vi "NXT-CAM-Remote.vi"() -> ()   [LabVIEW 2009]
uses:
  <vilib>/NXT/Subs/LVHSConnector.ctl
  <vilib>/NXT/Block Support/NXT_InputPort.ctl
  <vilib>/NXT/Dual Mode Library/Display/NXT_Rect.ctl
panel:
  in  "Tracking Mode":u8(ring) items=["Disable Tracking", "Get First Object", "Get n th Object", "Enable Tracking", "Sort Objects  by size", "Sort Objects  by Colors", "Illumination on ", "Illumination Off", "Write Colormap", "Read Colormap", "Line tracking mode", "Object Tracking mode"]
  in  "Object Number to Track":u8 format="%x"
  in  "Input Port":T1 caption="Port (Port 4)" items=["Port 1", "Port 2", "Port 3", "Port 4"]
  in  "Height":i32
  in  "Width":i32
  in  "Left":i32
  in  "Bottom":i32
  in  "NXT":T2={"error"={"status"=FALSE, "code"=0, "source"=""}, "address"="", "NXT #"=-1, "Show Error"=TRUE}
  out "Total Objects":u8=8
  out "X Upper Left":u8=108
  out "X Lower Right":u8=155
  out "Y Lower Right":u8=113
  out "Y Upper Left":u8=80
  out "Color":u8=1
  out "NXT dup":T2={"error"={"status"=FALSE, "code"=0, "source"=""}, "address"="", "NXT #"=-1, "Show Error"=TRUE} caption="NXT"
  out "Status \n(boolean)":bool
  # "mindsensors.com\nCopyright (c) 2009 by mindsensors.com\nEmail: info (<at>) mindsensors (<dot>) com\n\nThis program is free software. You can redistribute it and/or modify\nit under the terms of the GNU General Public License as published by\nthe Free Software Foundation; version 3 of the License.\nRead the license at: http://www.gnu.org/licenses/gpl.txt"
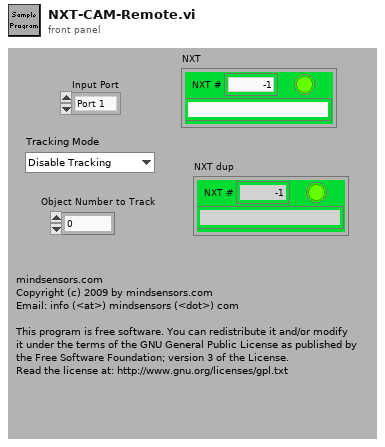
[diagram p1: front panel]
types:
  T1 = typedef "NXT_InputPort.ctl" = u8
  T2 = typedef "LVHSConnector.ctl" = cluster{"error":errorcluster, "address":string, "NXT #":i32, "Show Error":bool}
  T3 = typedef "NXT_Rect.ctl" = cluster{"Left":i16, "Bottom":i16, "Width":i16, "Height":i16}
  T4 = cluster{"Bottom":i32, "Left":i32, "Width":i32, "Height":i32}
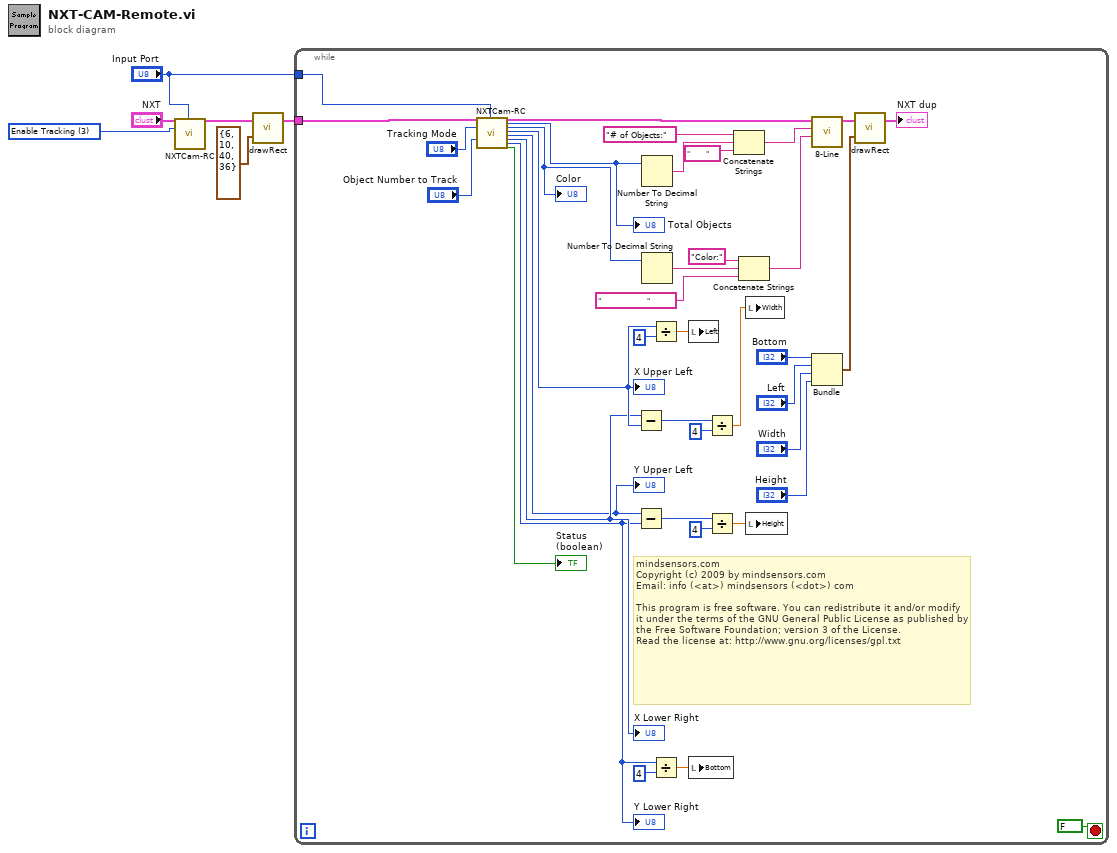
[diagram p0: block diagram]
diagram:
  w1 = u8 3 items=["Disable Tracking", "Get First Object", "Get n th Object", "Enable Tracking", "Sort Objects  by size", "Sort Objects  by Colors", "Illumination on ", "Illumination Off", "Write Colormap", "Read Colormap", "Line tracking mode", "Object Tracking mode"] ("Tracking Mode")
  n1 = call "NXTCam-RC.vi"("NXT"="NXT", "Tracking Mode"=w1, "Input Port"="Input Port") -> ("NXT dup"=w4:T2)  [unwired: 17 in, 7 out]
  n2 = call <vilib>:"drawRect.vi"("Rect Parameters"=T3 {"Left"=6, "Bottom"=10, "Width"=40, "Height"=36}, "NXT"=w4) -> ("NXT"=w3:T2)  [unwired: 2 in]
  n3 = while {
    tunnel: w3 -> [w44]
    tunnel: "Input Port" -> [w43]
    stop <- FALSE stop-if-true
    # "mindsensors.com\nCopyright (c) 2009 by mindsensors.com\nEmail: info (<at>) mindsensors (<dot>) com\n\nThis program is free software. You can redistribute it and/or modify\nit under the terms of the GNU General Public License as published by\nthe Free Software Foundation; version 3 of the License.\nRead the license at: http://www.gnu.org/licenses/gpl.txt"
    n4 = call "NXTCam-RC.vi"("NXT"=w44, "Tracking Mode"="Tracking Mode", "Object Number to Track"="Object Number to Track", "Input Port"=w43) -> ("NXT dup"=w19:T2, "Total Tracked Objects"=w15:u8, "Color"=w14:u8, "X Upper Left"=w13:u8, "Y Upper Left"=w11:u8, "X Lower Right"=w12:u8, "Y Lower Right"=w10:u8, "Status (boolean)"=→"Status \n(boolean)":bool)  [unwired: 16 in]
    "Total Objects" <- w15
    "X Upper Left" <- w13
    "X Lower Right" <- w12
    "Y Lower Right" <- w10
    "Y Upper Left" <- w11
    "Color" <- w14
    n5 = Subtract(x=w12, y=w13) -> (x-y=w23:u8)
    n6 = Subtract(x=w11, y=w10) -> (x-y=w20:u8)
    n7 = Number To Decimal String(number=w15) -> (decimal integer string=w37:string)  [unwired: 1 in]
    n8 = Number To Decimal String(number=w14) -> (decimal integer string=w39:string)  [unwired: 1 in]
    n9 = Divide(x=w13, y=4) -> (x/y=w26:dbl)
    n10 = Divide(x=w10, y=4) -> (x/y=w27:dbl)
    n11 = local write "Left"(w26) -> ()
    n12 = local write "Bottom"(w27) -> ()
    n13 = Divide(x=w23, y=4) -> (x/y=w22:dbl)
    n14 = Divide(x=w20, y=4) -> (x/y=w21:dbl)
    n15 = Concatenate Strings("# of Objects:" ("string"), w37, "        " ("string")) -> (w36:string)
    n16 = Concatenate Strings("Color:" ("string"), w39, "                       " ("string")) -> (w35:string)
    n17 = local write "Width"(w22) -> ()
    n18 = local write "Height"(w21) -> ()
    n19 = call "8-Line.vi"("Line 2"=w35, "Line 1"=w36, "NXT"=w19) -> ("NXT 2"=w18:T2)  [unwired: 8 in]
    n20 = Bundle("Bottom"="Bottom", "Left"="Left", "Width"="Width", "Height"="Height") -> (w34:T4)  [unwired: 1 in]
    n21 = call <vilib>:"drawRect.vi"("Rect Parameters"=w34, "NXT"=w18) -> ("NXT"=→"NXT dup":T2)  [unwired: 2 in]
  }
